vi "ConfigParams - Set - CAN.vi"(8 "error in (no error)":errorcluster, 9 "WritePeriod_ms":i32=5, 10 "BoxID":i32=1, 11 "Ethernet in":refnum<class "ENET_BS1201.lvclass">) -> (0 "error out":errorcluster, 3 "Ethernet out":refnum<class "ENET_BS1201.lvclass">)   [LabVIEW 2021, in "BS120x Driver.lvlib" / "ENET_BS1201.lvclass"]
uses:
  ENET_BS1201.lvclass
panel:
  # "[CAN]\nBoxID = 1\nWritePeriod_ms = 5"
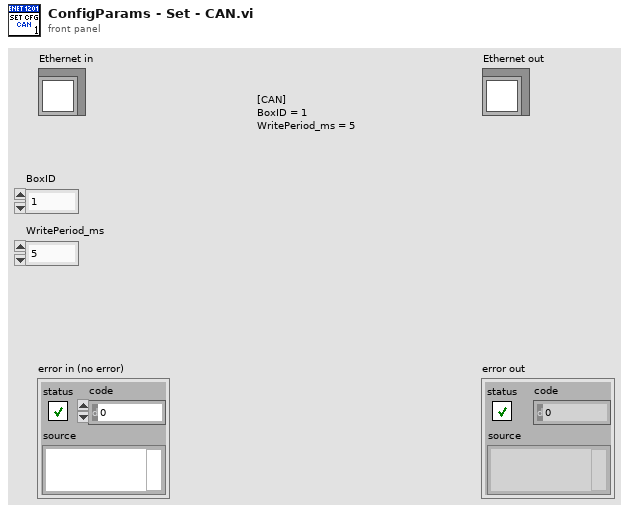
[diagram p1: front panel]
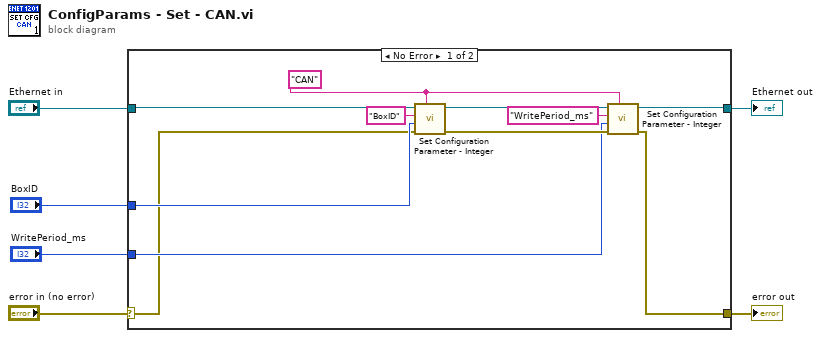
[diagram p0: block diagram]
diagram:
  n1 = case shown="No Error" "error in (no error)" {
    selector: "error in (no error)" -> [w7 w19]
    tunnel: [w9 w19] -> w5
    tunnel: [w10 w18] -> w3
    tunnel: "Ethernet in" -> [w8 w18]
    tunnel: "BoxID" -> [w16 _]
    tunnel: "WritePeriod_ms" -> [w11 _]
    frame No Error {
      w13 = "CAN" ("Section")
      n2 = call-dynamic "Set Configuration Parameter - Integer.vi"("Section"=w13, "error in (no error)"=w7, "Value"=w16, "Key"="BoxID", "Ethernet in"=w8) -> ("error out"=w14:errorcluster, "Ethernet out"=w15:refnum<class "ENET_BS1201.lvclass">)  [unwired: 5 in]
      n3 = call-dynamic "Set Configuration Parameter - Integer.vi"("Section"=w13, "error in (no error)"=w14, "Value"=w11, "Key"="WritePeriod_ms", "Ethernet in"=w15) -> ("error out"=w9:errorcluster, "Ethernet out"=w10:refnum<class "ENET_BS1201.lvclass">)  [unwired: 5 in]
    }
    frame Error {
    }
  }
  "error out" <- w5
  "Ethernet out" <- w3
